vi "PFI-28000-System_Reset System State.vi"(0 "PFI-28000-System in":refnum<class "PFI-28000-System.lvclass">, 11 "error in (no error)":errorcluster) -> (4 "PFI-28000-System out":refnum<class "PFI-28000-System.lvclass">, 15 "error out":errorcluster)   [LabVIEW 2017, in "PFI-28000-System.lvclass"]
uses:
  PFI-28000-System.lvclass
  C:/wc/07143 Precision Filters 28000 Support/Driver/source/Base/PFI-28000-Base.lvclass
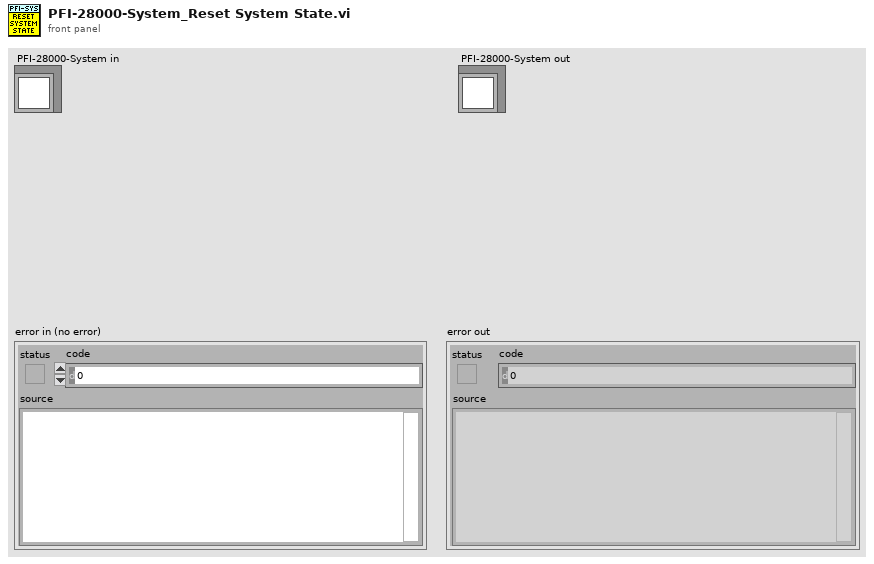
[diagram p1: front panel]
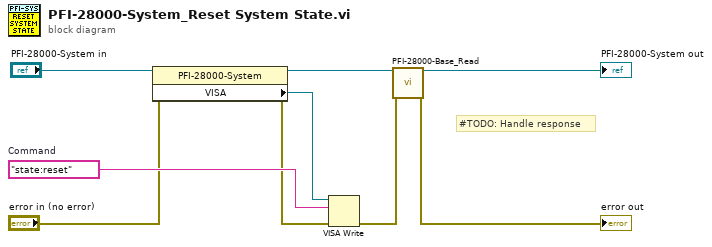
[diagram p0: block diagram]
diagram:
  w7 = "state:reset"  # Command
  # "#TODO: Handle response"
  n1 = property class="PFI-28000-System"(reference="PFI-28000-System in", error in="error in (no error)") -> (reference out=w4:refnum<class "PFI-28000-System.lvclass">, error out=w5:errorcluster, "VISA"=w8:refnum<visa-resource-name>)
  n2 = VISA Write(VISA resource name=w8, write buffer=w7, error in (no error)=w5) -> (error out=w2:errorcluster)  [unwired: 2 out]
  n3 = call-dynamic "PFI-28000-Base_Read.vi"("PFI-28000-Base in"=w4, "error in (no error)"=w2) -> ("PFI-28000-Base out"=→"PFI-28000-System out":refnum<class "PFI-28000-System.lvclass">, "error out"=→"error out":errorcluster)  [unwired: 10 in, 2 out]
